vi "data_entry_string.vi"(7 "caller":refnum<vi>, 8 "error in (no error)":errorcluster, 11 "configuration":T1={"dialog_text"="", "boolean_text_1"="", "boolean_text_2"="", "boolean_text_3"="", "inner_color"=16711680, "outer_color"=6618880, "wait_s"=nan, "error_status"=FALSE, "error_source"="", "error_details"="", "string []"=[], "custom_entry"=FALSE}) -> (0 "error out":errorcluster, 2 "data_entry out":string, 3 "dialog_selection":T2)   [LabVIEW 2015, in "lv-dialog-interfaces.lvlib"]
uses:
  lv-dialog-interfaces.lvlib
  lv-dialog/api/v1/public/_controls/dialog_selection.ctl
  lv-dialog/api/v1/public/_controls/configuration.ctl
  _controls/dialog_type.ctl
  _controls/hmi_references.ctl
  <vilib>/event_ctls.llb/eventvkey.ctl
  lv-dialog/api/v1/v1.lvlib
panel:
  out "dialog":string
  in  "data_entry":string
  in  "button 1":bool
  in  "button_2":bool
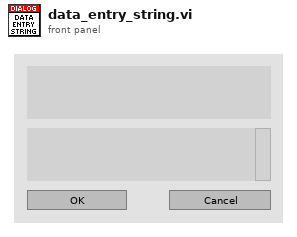
[diagram p1: front panel]
types:
  T1 = typedef "lv-dialog.lvlib/v1.lvlib/configuration.ctl" = cluster{"dialog_text":string, "boolean_text_1":string, "boolean_text_2":string, "boolean_text_3":string, "inner_color":u32, "outer_color":u32, "wait_s":dbl, "error_status":bool, "error_source":string, "error_details":string, "string []":string[], "custom_entry":bool}
  T2 = typedef "lv-dialog.lvlib/v1.lvlib/dialog_selection.ctl" = enum16{"null", "panel_closed", "button_1", "button_2", "button_3", "cancelled"}
  T3 = typedef "lv-dialog-interfaces.lvlib/dialog_type.ctl" = enum16{"null", "one_button", "two_button", "three_button", "confirmation", "busy_wait", "error", "busy_wait_embed", "combo_box", "data_entry_string", "data_entry_numeric"}
  T4 = typedef "lv-dialog-interfaces.lvlib/hmi_references.ctl" = cluster{"vi_reference":refnum<vi>, "caller":refnum<vi>, "dialog":refnum<vi>, "button_1":refnum<vi>, "button_2":refnum<vi>, "button_3":refnum<vi>, "busy":refnum<vi>, "error_glyph":refnum<vi>, "error_source":refnum<vi>, "error_text":refnum<vi>, "combo_box":refnum<vi>}
  T5 = typedef "eventvkey.ctl" = enum16{"ASCII", "Enter", "Return", "Shift", "Ctrl", "Alt", "Cmd", "Opt", "Caps", "NumLock", "Clear", "Break", "Up", "Down", "Left", "Right", "Insert", "Delete", "Home", "End", "PageUp", "PageDown", "Escape", "Help", "Pause", "ScrollLock", "F1", "F2", "F3", "F4", "F5", "F6", "F7", "F8", "F9", "F10", "F11", "F12", "F13", "F14", "F15", "F16", "F17", "F18", "F19", "F20", "F21", "F22", "F23", "F24", "Play", "VolumeUp", "VolumeDown", "Mute", "Two Byte Char"}
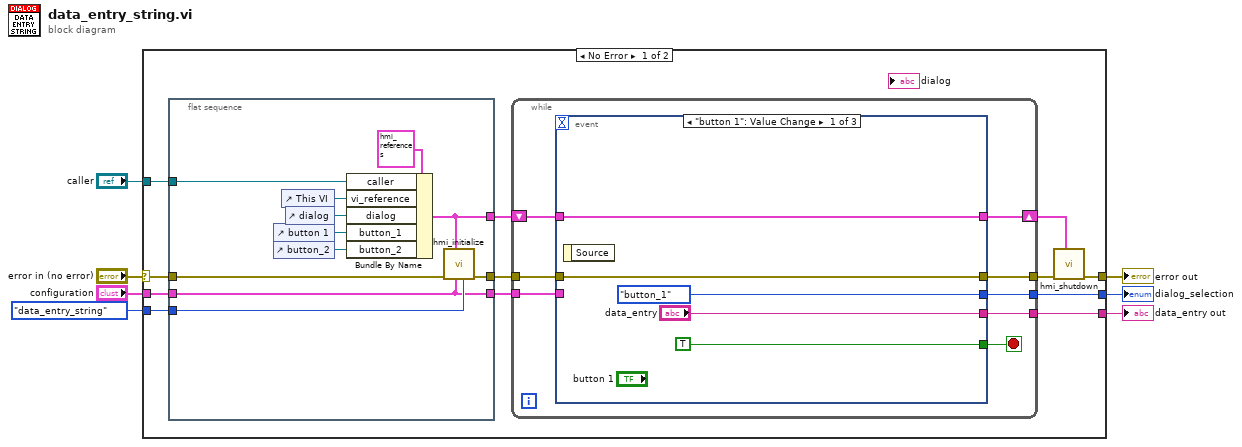
[diagram p0: block diagram]
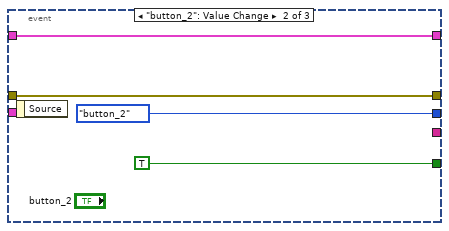
[diagram p2: hidden frame]
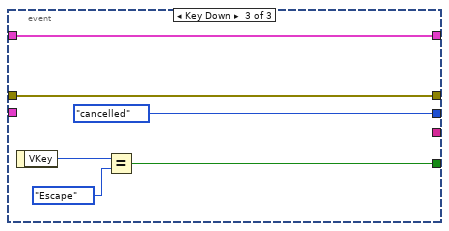
[diagram p3: hidden frame]
diagram:
  n1 = case shown="No Error" "error in (no error)" {
    selector: "error in (no error)" -> [w17 w54]
    tunnel: [w18 w54] -> w7
    tunnel: [w16 _] -> w5
    tunnel: "caller" -> [w15 _]
    tunnel: "configuration" -> [w14 _]
    tunnel: dialog_type."data_entry_string" ("dialog_type") -> [w13 _]
    tunnel: [w8 _] -> w1
    frame No Error {
      n2 = flat-sequence {
        tunnel: w17 -> [w23]
        tunnel: w14 -> [w20]
        tunnel: [w24] -> w12
        tunnel: [w20] -> w11
        tunnel: w15 -> [w28]
        tunnel: w13 -> [w22]
        tunnel: [w21] -> w10
        frame #0 {
          n3 = control-ref of="button 1"() -> (w27:refnum<vi>)
          n4 = control-ref of="button_2"() -> (w26:refnum<vi>)
          n5 = control-ref of="This VI"() -> (w29:refnum<vi>)
          n6 = control-ref of="dialog"() -> (w25:refnum<vi>)
          n7 = Bundle By Name(cluster=T4 {"vi_reference"=refnum, "caller"=refnum, "dialog"=refnum, "button_1"=refnum, "button_2"=refnum, "button_3"=refnum, "busy"=refnum, "error_glyph"=refnum, "error_source"=refnum, "error_text"=refnum, "combo_box"=refnum} ("references"), "caller"=w28, "vi_reference"=w29, "dialog"=w25, "button_1"=w27, "button_2"=w26) -> (w21:T4)
          n8 = call "hmi_initialize.vi"("dialog_type"=w22, "configuration"=w20, "references"=w21, "error in (no error)"=w23) -> ("error out"=w24:errorcluster)  [unwired: 7 in]
        }
      }
      n9 = while {
        tunnel: w12 -> [w35]
        tunnel: [w38] -> w16
        tunnel: w11 -> [w36]
        tunnel: [w34] -> w19
        shift-right: [w32] -> w9
        shift-left: w10 -> [w33]
        tunnel: [w31] -> w8
        stop <- w37 stop-if-true
        n10 = event shown="[0] \"button 1\": Value Change" {
          selector: _ -> [_ _ _]
          dyn-events: _ -> [_ _ _]
          timeout: _ -> [_ _ _]
          tunnel: [dialog_selection."button_1" ("dialog_selection") dialog_selection."button_2" ("dialog_selection") dialog_selection."cancelled" ("dialog_selection")] -> w38
          tunnel: [TRUE TRUE w50] -> w37
          tunnel: w36 -> [_ _ _]
          tunnel: w35 -> [w42 w45 w52]
          tunnel: [w42 w45 w52] -> w34
          tunnel: w33 -> [w40 w44 w51]
          tunnel: [w40 w44 w51] -> w32
          tunnel: ["data_entry" _ _] -> w31
          event "button 1": Value Change {
            n11 = event-data() -> ()  [unwired: 1 in, 1 out]
          }
          event "button_2": Value Change {
            n12 = event-data() -> ()  [unwired: 1 in, 1 out]
          }
          event Key Down {
            n13 = event-data() -> ("VKey"=w49:T5)  [unwired: 1 in]
            n14 = Equal?(x=w49, y=eventvkey."Escape" ("VKey")) -> (x = y?=w50:bool)
          }
        }
      }
      n15 = call "hmi_shutdown.vi"("references"=w9, "error in (no error)"=w19) -> ("error out"=w18:errorcluster)  [unwired: 9 in]
    }
    frame Error {
    }
  }
  "error out" <- w7
  "dialog_selection" <- w5
  "data_entry out" <- w1
